vi "GetDBPath.vi"(1 "Filename":string) -> (0 "Connection":string)   [LabVIEW 2014]
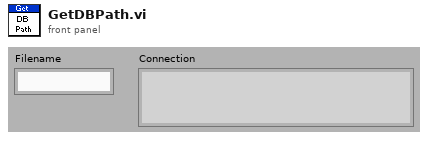
[diagram p1: front panel]
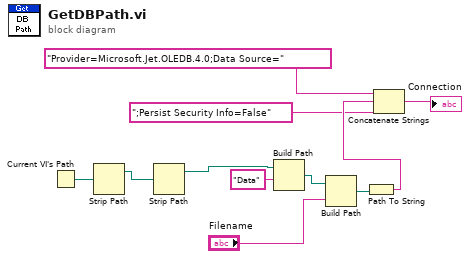
[diagram p0: block diagram]
diagram:
  n1 = Current VI's Path() -> (path=w3:path)
  n2 = Strip Path(path=w3) -> (stripped path=w2:path)  [unwired: 1 out]
  n3 = Strip Path(path=w2) -> (stripped path=w1:path)  [unwired: 1 out]
  n4 = Build Path(base path=w1, name or relative path="Data") -> (appended path=w11:path)
  n5 = Build Path(base path=w11, name or relative path="Filename") -> (appended path=w8:path)
  n6 = Path To String(path=w8) -> (string=w7:string)
  n7 = Concatenate Strings("Provider=Microsoft.Jet.OLEDB.4.0;Data Source=" ("string"), w7, ";Persist Security Info=False" ("string")) -> (→"Connection":string)
